vi "getStageXML.vi"(8 "error in (no error)":errorcluster, 11 "ScriptEvent in":refnum<class "ScriptEvent.lvclass">) -> (0 "error out":errorcluster, 2 "stageXML":refnum<class "xmlNode.lvclass">, 3 "ScriptEvent out":refnum<class "ScriptEvent.lvclass">)   [LabVIEW 2009, in "Tools.lvlib" / "Scripting.lvlib" / "ScriptEvent.lvclass"]
uses:
  ScriptEvent.lvclass
  xmlNode/xmlNode.lvclass
  ScriptEvent.lvclass/ScriptEvent.ctl
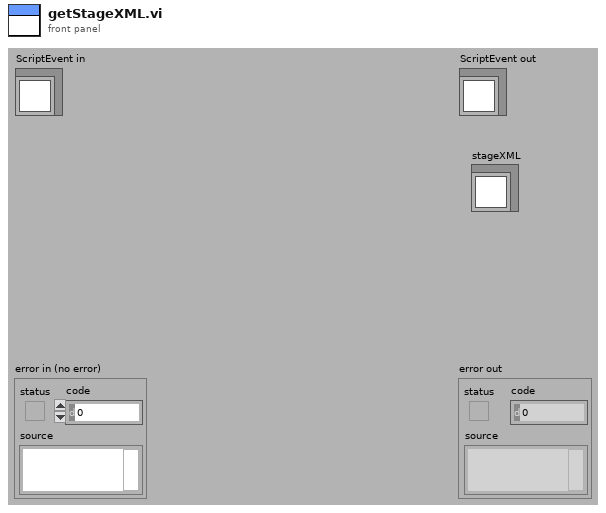
[diagram p1: front panel]
types:
  T1 = enum16{"Initialise", "MOT", "Molasses", "Optical Pumping", "Magnetic Trap", "RF Cooling", "Manipulation", "Switch Off", "Absorption Imaging", "Fluorscence Imaging", "Shut Down"}
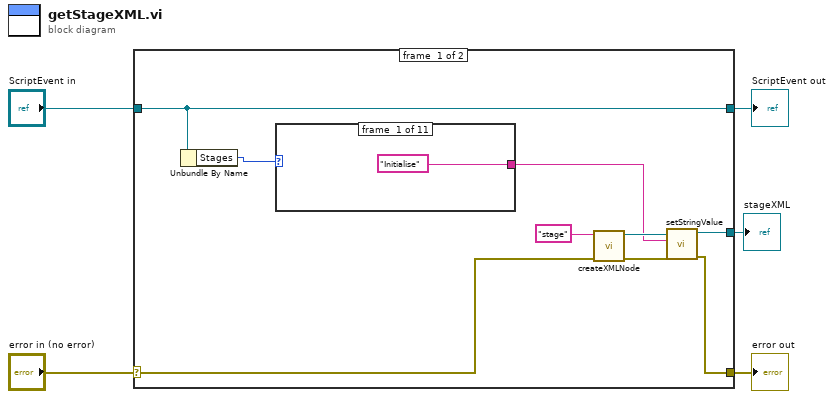
[diagram p0: block diagram]
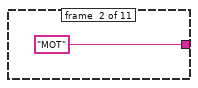
[diagram p2: hidden frame]
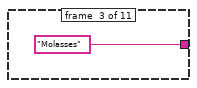
[diagram p3: hidden frame]
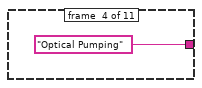
[diagram p4: hidden frame]
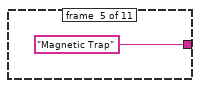
[diagram p5: hidden frame]
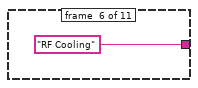
[diagram p6: hidden frame]
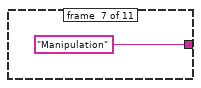
[diagram p7: hidden frame]
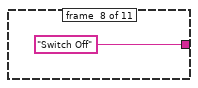
[diagram p8: hidden frame]
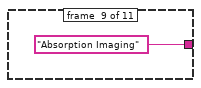
[diagram p9: hidden frame]
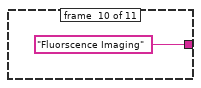
[diagram p10: hidden frame]
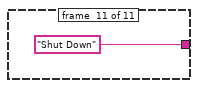
[diagram p11: hidden frame]
diagram:
  n1 = case shown="No Error" "error in (no error)" {
    selector: "error in (no error)" -> [w9 w27]
    tunnel: [w10 w27] -> w4
    tunnel: [w8 w26] -> w2
    tunnel: "ScriptEvent in" -> [w8 w26]
    tunnel: [w11 _] -> w1
    frame #0 {
      n2 = Unbundle By Name(w8) -> ("Stages"=w7:T1)
      n3 = case shown="\"Molasses\"" w7 {
        tunnel: ["Initialise" "MOT" "Molasses" "Optical Pumping" "Magnetic Trap" "RF Cooling" "Manipulation" "Switch Off" "Absorption Imaging" "Fluorscence Imaging" "Shut Down"] -> w6
        frame #0 {
        }
        frame #1 {
        }
        frame #2 {
        }
        frame #3 {
        }
        frame #4 {
        }
        frame #5 {
        }
        frame #6 {
        }
        frame #7 {
        }
        frame #8 {
        }
        frame #9 {
        }
        frame #10 {
        }
      }
      n4 = call "createXMLNode.vi"("error in (no error)"=w9, "name"="stage") -> ("error out"=w12:errorcluster, "xmlNode out"=w13:refnum<class "xmlNode.lvclass">)  [unwired: 8 in]
      n5 = call-dynamic "setStringValue.vi"("error in (no error)"=w12, "stringValue"=w6, "xmlNode.lvclass in"=w13) -> ("error out"=w10:errorcluster, "xmlNode.lvclass out"=w11:refnum<class "xmlNode.lvclass">)  [unwired: 7 in]
    }
    frame #1 {
    }
  }
  "error out" <- w4
  "ScriptEvent out" <- w2
  "stageXML" <- w1
